vi "test_can.vi"() -> ()   [LabVIEW 2014]
panel:
  out "CloseDevice_Success?":u32
  in  "VCI_CAN_OBJ 2":T1={"ID"=0, "TimeStamp"=0, "TimeFlag"=0, "SendType"=2, "RemoteFlag"=0, "ExternFlag"=0, "DataLen"=8, "Data 0"=0, "Data 1"=1, "Data 2"=2, "Data 3"=3, "Data 4"=0, "Data 5"=0, "Data 6"=0, "Data 7"=0, "Reserved 0"=0, "Reserved 1"=0, "Reserved 2"=0}
  out "发送的帧数":u32=1
  out "VCI_CAN_OBJ":T1
  out "接收的帧数":u32=1
  in  "停止":bool
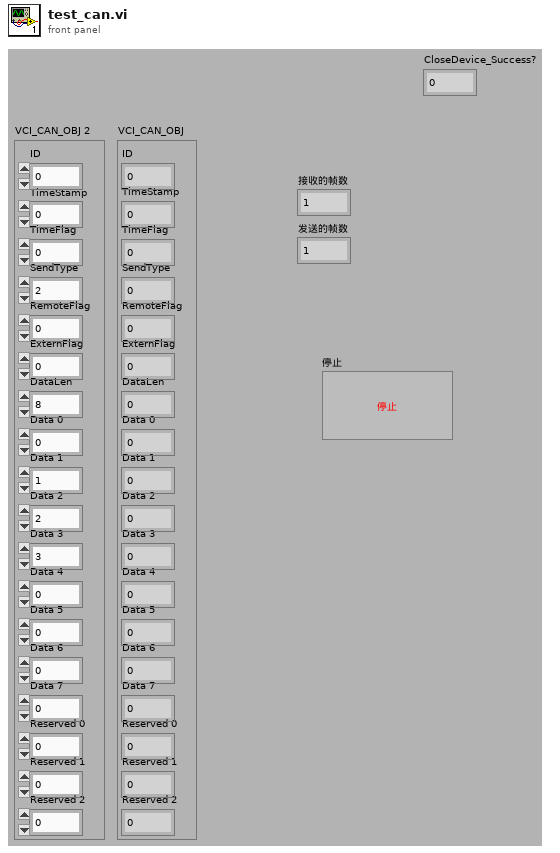
[diagram p1: front panel]
types:
  T1 = cluster{"ID":u32, "TimeStamp":u32, "TimeFlag":u8, "SendType":u8, "RemoteFlag":u8, "ExternFlag":u8, "DataLen":u8, "Data 0":u8, "Data 1":u8, "Data 2":u8, "Data 3":u8, "Data 4":u8, "Data 5":u8, "Data 6":u8, "Data 7":u8, "Reserved 0":u8, "Reserved 1":u8, "Reserved 2":u8}
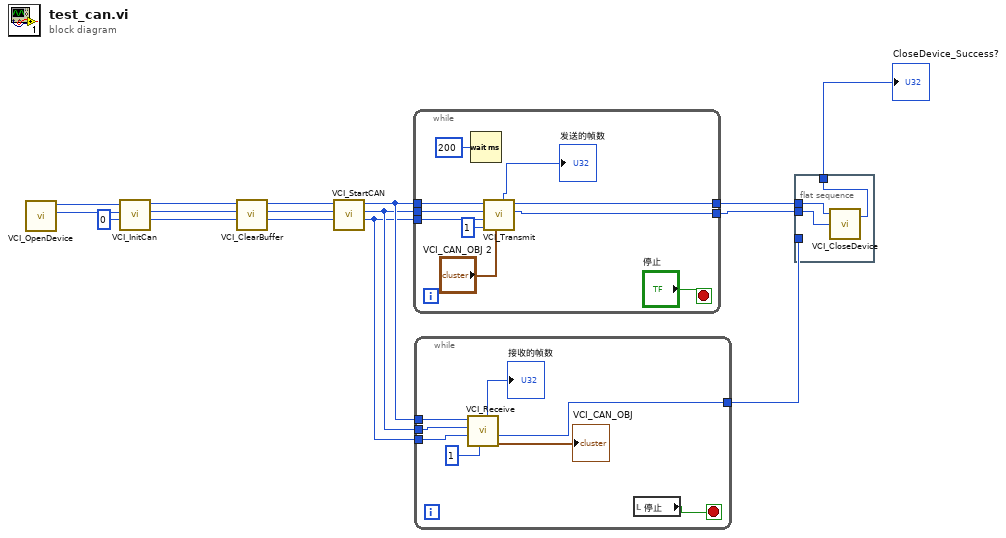
[diagram p0: block diagram]
diagram:
  n1 = call "VCI_OpenDevice.vi"() -> ("DevIndex"=w15:u32, "DevType"=w16:u32)  [unwired: 10 out]
  n2 = call "VCI_InitCan.vi"("CanIndex_IN"=u32 0, "DevIndex_IN"=w15, "DevType_IN"=w16) -> ("CanIndex_OUT"=w8:u32, "DevIndex_OUT"=w9:u32, "DevType_OUT"=w10:u32)  [unwired: 1 in, 5 out]
  n3 = call "VCI_ClearBuffer.vi"("CANIndex 2"=w8, "DevIndex 2"=w9, "DevType 2"=w10) -> ("CANIndex"=w5:u32, "DevIndex"=w6:u32, "DevType"=w7:u32)  [unwired: 6 out]
  n4 = call "VCI_StartCAN.vi"("CANIndex"=w5, "DevIndex"=w6, "DevType"=w7) -> ("CANIndex 2"=w11:u32, "DevIndex 2"=w12:u32, "DevType 2"=w13:u32)  [unwired: 6 out]
  n5 = while {
    tunnel: w13 -> [w26]
    tunnel: w12 -> [w25]
    tunnel: w11 -> [w24]
    tunnel: [w18] -> w4
    tunnel: [w17] -> w3
    stop <- "停止" stop-if-true
    n6 = Wait (ms)(milliseconds to wait=u32 200 ("等待时间（毫秒）")) -> ()  [unwired: 1 out]
    n7 = call "VCI_Transmit.vi"("VCI_CAN_OBJ"="VCI_CAN_OBJ 2", "Len"=u32 1, "CANIndex"=w24, "DevIndex"=w25, "DevType"=w26) -> ("DevIndex 2"=w17:u32, "DevType 2"=w18:u32, "发送的帧数"=→"发送的帧数":u32)  [unwired: 4 out]
  }
  n8 = while {
    tunnel: w13 -> [w34]
    tunnel: w12 -> [w33]
    tunnel: w11 -> [w32]
    tunnel: [w27] -> w1
    stop <- w28 stop-if-true
    n9 = call "VCI_Receive.vi"("Len"=u32 1, "CANIndex"=w32, "DevIndex"=w33, "DevType"=w34) -> ("VCI_CAN_OBJ"=→"VCI_CAN_OBJ":T1, "CANIndex 2"=w27:u32, "接收的帧数"=→"接收的帧数":u32)  [unwired: 1 in, 4 out]
    n10 = local read "停止"() -> (w28:bool)
  }
  n11 = flat-sequence {
    tunnel: w4 -> [w37]
    tunnel: w3 -> [w36]
    tunnel: [w35] -> w2
    tunnel: w1 -> [_]
    frame #0 {
      n12 = call "VCI_CloseDevice.vi"("DevIndex"=w36, "DevType"=w37) -> ("CloseDevice_Success?"=w35:u32)  [unwired: 1 in, 1 out]
    }
  }
  "CloseDevice_Success?" <- w2
